vi "configureAutoExposure.vi"(0 "Camera in":refnum<class "Camera.lvclass">, 1 "region_type":u16(ring) items=["balanced", "center_based", "corner_based", "full"], 2 "min_exposure_s":dbl=0.001, 3 "max_exposure_s":dbl=0.1, 5 "error in (no error)":errorcluster) -> (14 "Camera out":refnum<class "Camera.lvclass">, 19 "error out":errorcluster)   [LabVIEW 2019, in "Camera.lvclass"]
doc: "Configures the auto exposure parameters\n\nThis does not (de)activate the auto exposure functionality, \ntherefore use autoExposureOn.vi and autoExposureOff.vi"
uses:
  Camera.lvclass
  Camera.lvclass/Camera.ctl
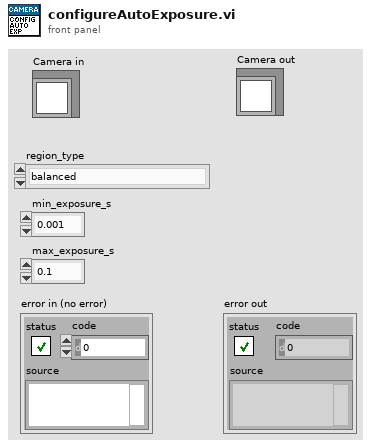
[diagram p1: front panel]
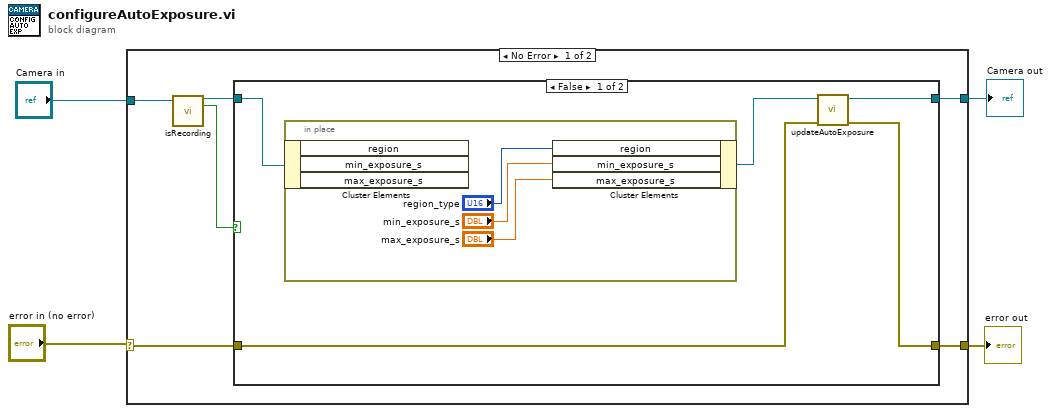
[diagram p0: block diagram]
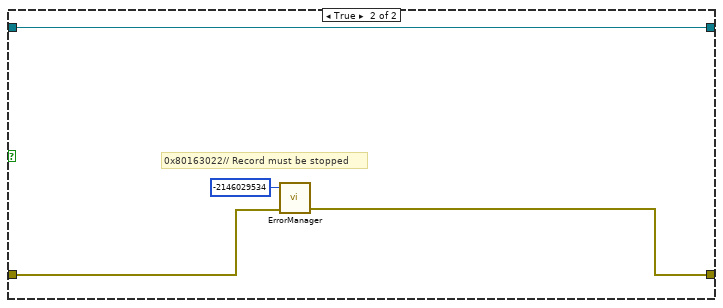
[diagram p2: hidden frame]
diagram:
  n1 = case shown="No Error" "error in (no error)" {
    selector: "error in (no error)" -> [w6 w24]
    tunnel: [w5 w24] -> w3
    tunnel: "Camera in" -> [w10 w23]
    tunnel: [w7 w23] -> w1
    frame No Error {
      n2 = call-dynamic "isRecording.vi"("Camera in"=w10) -> ("Camera out"=w8:refnum<class "Camera.lvclass">, "recording"=w9:bool)  [unwired: 12 in, 1 out]
      n3 = case shown="False" w9 {
        tunnel: w8 -> [w15 w22]
        tunnel: [w13 w22] -> w7
        tunnel: w6 -> [w12 w21]
        tunnel: [w11 w19] -> w5
        frame False {
          n4 = in-place {
            n5 = in-place-cluster #1(w15) -> ()  [unwired: 3 out]
            n6 = in-place-cluster #1("region"="region_type", "min_exposure_s"="min_exposure_s", "max_exposure_s"="max_exposure_s") -> (w14:refnum<class "Camera.lvclass">)
          }
          n7 = call "updateAutoExposure.vi"("error in (no error)"=w12, "Camera in"=w14) -> ("error out"=w11:errorcluster, "Camera out"=w13:refnum<class "Camera.lvclass">)  [unwired: 8 in]
        }
        frame True {
          # "0x80163022// Record must be stopped"
          n8 = call "ErrorManager.vi"("error in (no error)"=w21, "error code"=-2146029534) -> ("error out"=w19:errorcluster)  [unwired: 2 in, 1 out]
        }
      }
    }
    frame Error {
    }
  }
  "error out" <- w3
  "Camera out" <- w1
